vi "AdjustMaxMin.vi"(3 "Max In":dbl format="%#_13g", 4 "Min In":dbl format="%#_13g", 6 "Input":dbl format="%#_13g") -> (0 "Max Out":dbl format="%#_13g", 1 "Min Out":dbl format="%#_13g", 5 "Bounds Extended":bool)   [LabVIEW 2016]
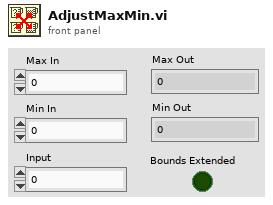
[diagram p1: front panel]
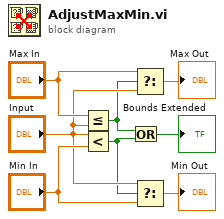
[diagram p0: block diagram]
diagram:
  n1 = Less Or Equal?(x="Max In", y="Input") -> (x <= y?=w1:bool)
  n2 = Less?(x="Input", y="Min In") -> (x < y?=w2:bool)
  n3 = Or(x=w1, y=w2) -> (x .or. y?=→"Bounds Extended":bool)
  n4 = Select(t="Max In", s=w1, f="Input") -> (s? t:f=→"Max Out":dbl)
  n5 = Select(t="Input", s=w2, f="Min In") -> (s? t:f=→"Min Out":dbl)
